vi "显示JPEG图片.vi"(1 "图片":string, 2 "AppData路径":path) -> (0 "二维图片":picture)   [LabVIEW 2018]
uses:
  <vilib>/picture/picture.llb/Draw True-Color Pixmap.vi
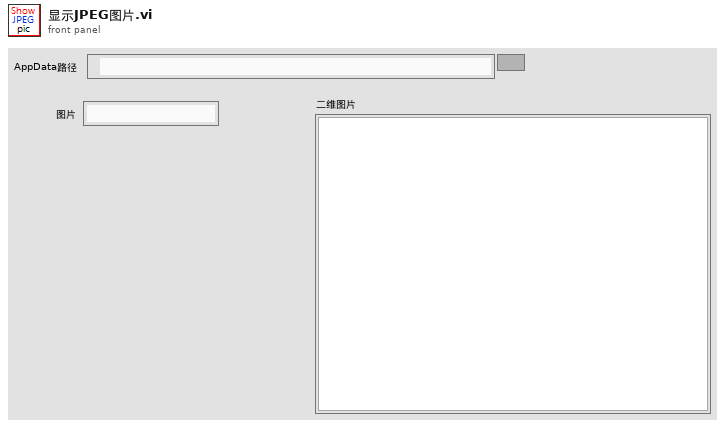
[diagram p1: front panel]
types:
  T1 = typedef "imagedata.ctl" = cluster{"image type":i32, "image depth":i32, "image":u8[], "mask":u8[], "colors":u32[], "Rectangle":cluster{"left":i16, "top":i16, "right":i16, "bottom":i16}}
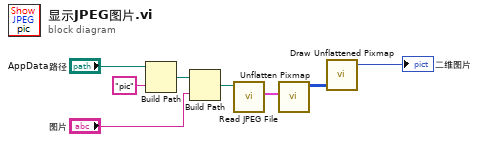
[diagram p0: block diagram]
diagram:
  n1 = Build Path(base path="AppData路径", name or relative path="pic" ("名称或相对路径")) -> (appended path=w3:path)
  n2 = Build Path(base path=w3, name or relative path="图片") -> (appended path=w2:path)
  n3 = call <vilib>:"Read JPEG File.vi"("path to JPEG file"=w2) -> ("image data"=w6:T1)  [unwired: 8 in, 2 out]
  n4 = call <vilib>:"Unflatten Pixmap.vi"("image data"=w6) -> ("24-bit pixmap"=w7:u32[][])  [unwired: 4 in, 6 out]
  n5 = call-poly <vilib>:"Draw Unflattened Pixmap.vi"("data (RGB format)"=w7) -> ("new picture"=→"二维图片":picture)  [unwired: 8 in]
